vi "Globale Variable.vi"() -> ()   [LabVIEW 2016]
panel:
  out "manual Gain":bool
  out "lc":bool
  out "voltage_start":dbl
  out "starting threshhold":dbl
  out "v_max":dbl
  out "lambda_target":dbl
  out "am":bool
  out "lambda error":dbl
  out "vHL":dbl
  out "vHR":dbl
  out "throttle voltage":dbl
  out "k_lqr":dbl
  out "lambda":dbl
  out "vVL":dbl
  out "v_rear":dbl
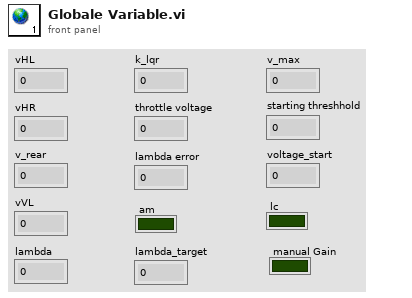
[diagram p1: front panel]
diagram:
